vi "test.vi"() -> ()   [LabVIEW 2023]
uses:
  tajmer_kontrola.ctl
panel:
  in  "Vrijeme od kog se broji":dbl
  out "Status":T1
  out "error out":errorcluster
  in  "error in (no error)":errorcluster
  in  "Enum":T2
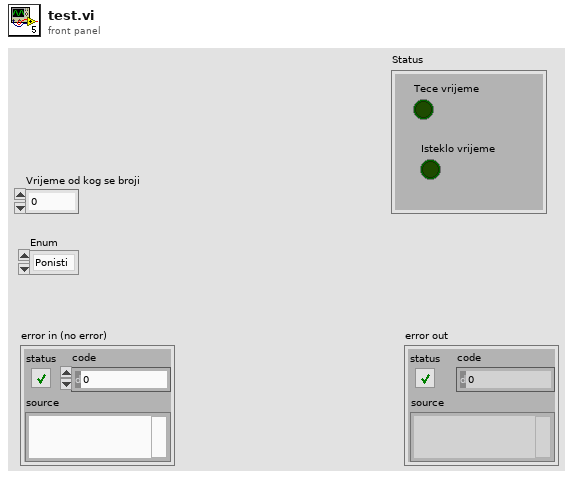
[diagram p1: front panel]
types:
  T1 = cluster{"Tece vrijeme":bool, "Isteklo vrijeme":bool}
  T2 = typedef "tajmer_kontrola.ctl" = enum16{"Ponisti", "Provjeri"}
  T3 = cluster{"Poslednje ocitano vrijeme":dbl, "Proteklo vrijeme":dbl}
  T4 = cluster{"Vrijeme tece":bool, "Isteklo vrijeme":bool}
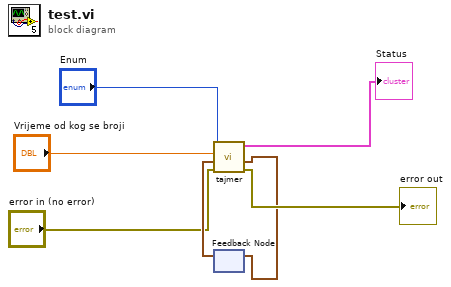
[diagram p0: block diagram]
diagram:
  n1 = feedback #1() -> (w7:T3)  [unwired: 1 in]
  n2 = call "tajmer.vi"("error in (no error)"="error in (no error)", "ulazni podaci tajmera"=w7, "Vrijeme od kog se broji"="Vrijeme od kog se broji", "Enum"="Enum") -> ("error out"=→"error out":errorcluster, "izlazni podaci tajmera"=w1:T3, "status tajmera"=→"Status":T4)  [unwired: 5 in]
  n3 = feedback-in #1(w1) -> ()
